vi "Get Connections - NPin MConn.vi"(6 "pin type":T3, 8 "error in":errorcluster, 9 "site":i32, 10 "pin or relay names":string[](array[string]), 11 "session reservation in":refnum<class "Session Reservation.lvclass">) -> (0 "error out":errorcluster, 2 "connections":T1[](array[typedef]), 3 "session reservation out":refnum<class "Session Reservation.lvclass">)   [LabVIEW 2021, in "Session Management niDAQmx.lvlib"]
uses:
  Session Management niDAQmx.lvlib
  <vilib>/Plug-In SDKs/Clients/Session Management V1/Session Reservation/Pin Type.ctl
  <vilib>/Plug-In SDKs/Clients/Session Management V1/Session Reservation/Session Reservation.lvclass
  Connection with Session.ctl
  Session Factory/Session Factory.lvclass
  C:/Program Files/National Instruments/LabVIEW 2021/vi.lib/Plug-In SDKs/Sessions/Instrument/ISession Factory/ISession Factory.lvclass
  <vilib>/Plug-In SDKs/Clients/Session Management V1/Session Reservation/Connection.ctl
  7d89c178-3406-49cc-9d81-7ef77104617b.vi
  <vilib>/Plug-In SDKs/Clients/Session Management V1/Session Reservation/Get Connections Impl.vi
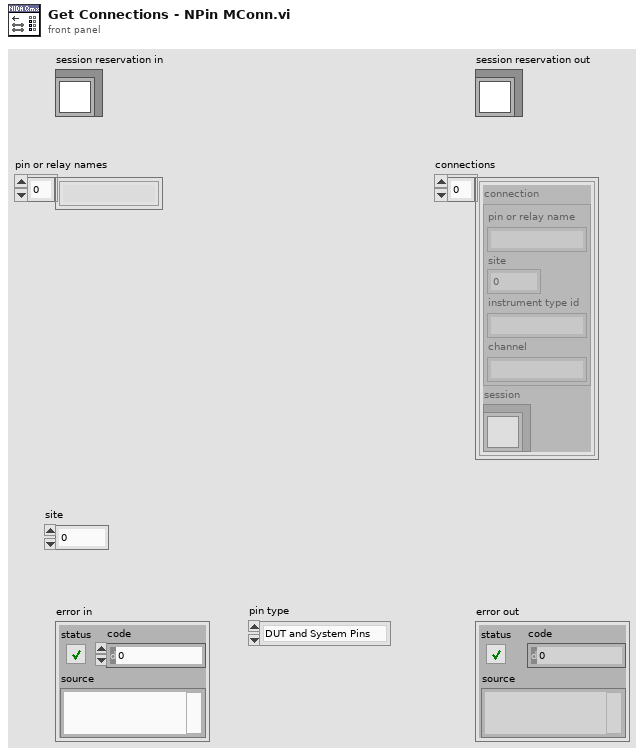
[diagram p1: front panel]
types:
  T1 = typedef "Session Management niDAQmx.lvlib/Connection with Session.ctl" = cluster{"connection":T2, "session":refnum<class "Session Factory.lvclass">}
  T2 = typedef "NI Session Management V1 Client.lvlib/Session Reservation.lvclass/Connection.ctl" = cluster{"pin or relay name":string, "site":i32, "instrument type id":string, "channel":string}
  T3 = typedef "NI Session Management V1 Client.lvlib/Session Reservation.lvclass/Pin Type.ctl" = enum16{"DUT and System Pins", "System Pins"}
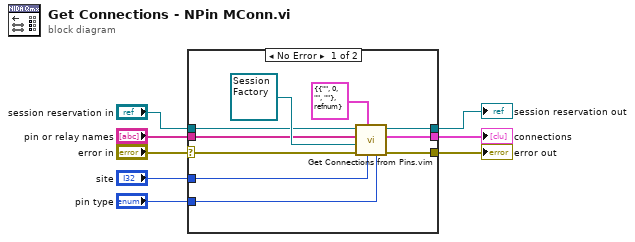
[diagram p0: block diagram]
diagram:
  n1 = case shown="No Error" "error in" {
    selector: "error in" -> [w18 w20]
    tunnel: "site" -> [w11 _]
    tunnel: "pin type" -> [w10 _]
    tunnel: [w17 w20] -> w5
    tunnel: "session reservation in" -> [w13 w19]
    tunnel: [w14 w19] -> w3
    tunnel: [w15 _] -> w2
    tunnel: "pin or relay names" -> [w9 _]
    frame No Error {
      n2 = call "Get Connections from Pins.vim"("pin type"=w10, "site"=w11, "connection type"=T1 {"connection"={"pin or relay name"="", "site"=0, "instrument type id"="", "channel"=""}, "session"=refnum} ("connection with task"), "error in"=w18, "session factory"=refnum<class "Session Factory.lvclass"> refnum ("Session Management niDAQmx.lvlib:Session Factory.lvclass"), "pin or relay names"=w9, "session reservation in"=w13) -> ("error out"=w17:errorcluster, "connections"=w15:T1[], "session reservation out"=w14:refnum<class "Session Reservation.lvclass">)  [unwired: 2 in]
    }
    frame Error {
    }
  }
  "error out" <- w5
  "session reservation out" <- w3
  "connections" <- w2
